vi "Register-events.vi"(8 "error in (no error)":errorcluster, 11 "Data ref. in":refnum<data-value>) -> (0 "error out":errorcluster, 1 "Events":refnum<event-registration>, 3 "Data ref.":refnum<data-value>)   [LabVIEW 2013, in "CameraVision.lvlib" / "CV-Main.lvclass"]
uses:
  CV-Main.lvclass
  CV-Main.lvclass/CV-Main.ctl
  Errors/CV-Errors.lvclass/CV-Errors.ctl
  Read Errors.vi
  Errors/Read Error event.vi
  Errors/CV-Errors.lvclass
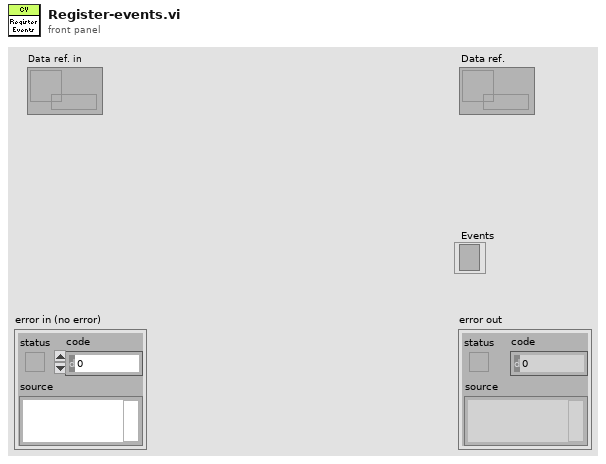
[diagram p1: front panel]
types:
  T1 = typedef "CameraVision.lvlib/CV-Errors.lvclass/Object-reference.ctl" = refnum<data-value>
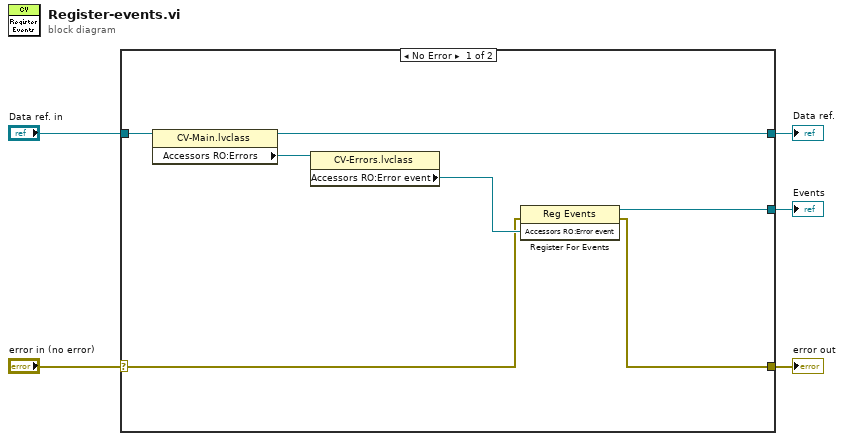
[diagram p0: block diagram]
diagram:
  n1 = case shown="No Error" "error in (no error)" {
    selector: "error in (no error)" -> [w8 w14]
    tunnel: [w7 w14] -> w4
    tunnel: "Data ref. in" -> [w12 w13]
    tunnel: [w11 w13] -> w2
    tunnel: [w6 _] -> w1
    frame No Error {
      n2 = property class="CV-Main.lvclass"(reference=w12) -> (reference out=w11:refnum<data-value>, "Accessors RO:Errors"=w10:T1)  [unwired: 1 in, 1 out]
      n3 = property class="CV-Errors.lvclass"(reference=w10) -> ("Accessors RO:Error event"=w9:refnum<user-event>)  [unwired: 1 in, 2 out]
      n4 = register-events(error in=w8, w9) -> (reference out=w6:refnum<event-registration>, error out=w7:errorcluster)  [unwired: 1 in]
    }
    frame Error {
    }
  }
  "error out" <- w4
  "Data ref." <- w2
  "Events" <- w1
